vi "Paint_Finded_Particles(X,Y)6.vi"(2 "error IN":errorcluster, 3 "Color":u32(colorbox)=16711680, 4 "Array of Points IN":dbl[](array[numeric]), 5 "Image IN":T1) -> (0 "error OUT":errorcluster, 1 "Image OUT":T1)   [LabVIEW 2013]
uses:
  <vilib>/vision/Image Controls.llb/IMAQ Image.ctl
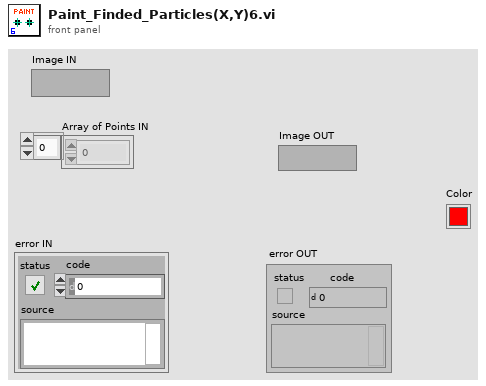
[diagram p1: front panel]
types:
  T1 = typedef "IMAQ Image.ctl" = refnum<image>
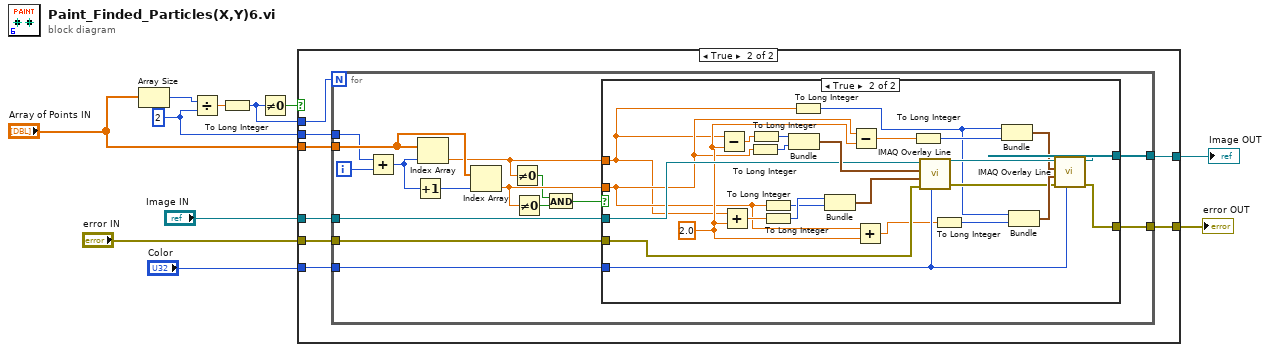
[diagram p0: block diagram]
diagram:
  w1 = 2 ("y")
  n1 = Array Size(array="Array of Points IN") -> (size(s)=w11:i32)
  n2 = Divide(x=w11, y=w1) -> (x/y=w5:dbl)
  n3 = To Long Integer(number=w5) -> (32bit integer=w3:i32)
  n4 = Not Equal To 0?(x=w3) -> (x != 0?=w4:bool)
  n5 = case shown="True" w4 {
    tunnel: "Image IN" -> [w13 w21]
    tunnel: "Array of Points IN" -> [_ w20]
    tunnel: "error IN" -> [w12 w19]
    tunnel: [w13 w18] -> w7
    tunnel: [w12 w17] -> w6
    tunnel: w3 -> [_ w16]
    tunnel: "Color" -> [_ w15]
    tunnel: w1 -> [_ w14]
    frame False {
    }
    frame True {
      n6 = for {
        N: w16 -> [_]
        tunnel: w21 -> [w32]
        tunnel: w20 -> [w36]
        tunnel: w19 -> [w33]
        tunnel: [w35] -> w18
        tunnel: [w34] -> w17
        tunnel: w15 -> [w31]
        tunnel: w14 -> [w24]
        i -> [w25]
        n7 = Add(x=w24, y=w25) -> (x+y=w23:i32)
        n8 = Increment(x=w23) -> (x+1=w22:i32)
        n9 = Index Array(array=w36, index=w23) -> (element=w30:dbl)
        n10 = Index Array(array=w36, index=w22) -> (element=w29:dbl)
        n11 = Not Equal To 0?(x=w30) -> (x != 0?=w27:bool)
        n12 = Not Equal To 0?(x=w29) -> (x != 0?=w28:bool)
        n13 = And(x=w27, y=w28) -> (x .and. y?=w26:bool)
        n14 = case shown="True" w26 {
          tunnel: w30 -> [_ w42]
          tunnel: w29 -> [_ w46]
          tunnel: [w38 w57] -> w35
          tunnel: [w37 w56] -> w34
          tunnel: w33 -> [w37 w55]
          tunnel: w32 -> [w38 w54]
          tunnel: w31 -> [_ w52]
          frame False {
          }
          frame True {
            w53 = 2.0 ("y")
            n15 = Subtract(x=w42, y=w53) -> (x-y=w48:dbl)
            n16 = Add(x=w42, y=w53) -> (x+y=w51:dbl)
            n17 = To Long Integer(number=w46) -> (32bit integer=w45:i32)
            n18 = To Long Integer(number=w48) -> (32bit integer=w47:i32)
            n19 = To Long Integer(number=w46) -> (32bit integer=w49:i32)
            n20 = To Long Integer(number=w51) -> (32bit integer=w50:i32)
            n21 = Bundle(w47, w45) -> (w61:cluster{i32, i32})  [unwired: 1 in]
            n22 = To Long Integer(number=w42) -> (32bit integer=w41:i32)
            n23 = Bundle(w50, w49) -> (w63:cluster{i32, i32})  [unwired: 1 in]
            n24 = Subtract(x=w46, y=w53) -> (x-y=w44:dbl)
            n25 = Add(x=w46, y=w53) -> (x+y=w40:dbl)
            n26 = To Long Integer(number=w44) -> (32bit integer=w43:i32)
            n27 = call "IMAQ Overlay Line"("Color"=w52, "error in (no error)"=w55, "End Point"=w63, "Start Point"=w61, "Image"=w54) -> ("error out"=w58:errorcluster, "Image Out"=w62:T1)  [unwired: 5 in]
            n28 = To Long Integer(number=w40) -> (32bit integer=w39:i32)
            n29 = Bundle(w41, w43) -> (w60:cluster{i32, i32})  [unwired: 1 in]
            n30 = Bundle(w41, w39) -> (w59:cluster{i32, i32})  [unwired: 1 in]
            n31 = call "IMAQ Overlay Line"("Color"=w52, "error in (no error)"=w58, "End Point"=w59, "Start Point"=w60, "Image"=w62) -> ("error out"=w56:errorcluster, "Image Out"=w57:T1)  [unwired: 5 in]
          }
        }
      }
    }
  }
  "Image OUT" <- w7
  "error OUT" <- w6
